vi "Read.vi"(8 "error in (no error)":errorcluster, 9 "Timeout":u32, 10 "Last message":refnum<class "BaseMessage.lvclass">, 11 "StringReader in":refnum<class "StringReader.lvclass">) -> (0 "error out":errorcluster, 1 "isAck?":bool, 2 "Responses":T1[](array[typedef]), 3 "StringReader out":refnum<class "StringReader.lvclass">)   [LabVIEW 2013, in "StringReader.lvclass"]
doc: "Read a message from the remote destination"
uses:
  StringReader.lvclass
  Message/BaseMessage/BaseMessage.lvclass
  response.ctl
  driver_status.ctl
  <vilib>/Utility/error.llb/whitespace.ctl
  StringReader.lvclass/StringReader.ctl
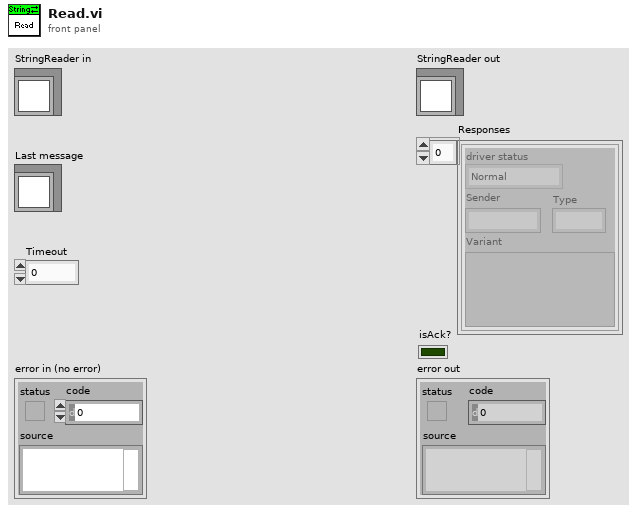
[diagram p1: front panel]
types:
  T1 = typedef "response.ctl" = cluster{"driver status":T2, "Sender":string, "Type":i32, "Variant":variant}
  T2 = typedef "driver_status.ctl" = enum16{"Normal", "Startup", "Connection lost", "Reconnected", "Timeout", "Idle", "Busy"}
  T3 = typedef "whitespace.ctl" = u16
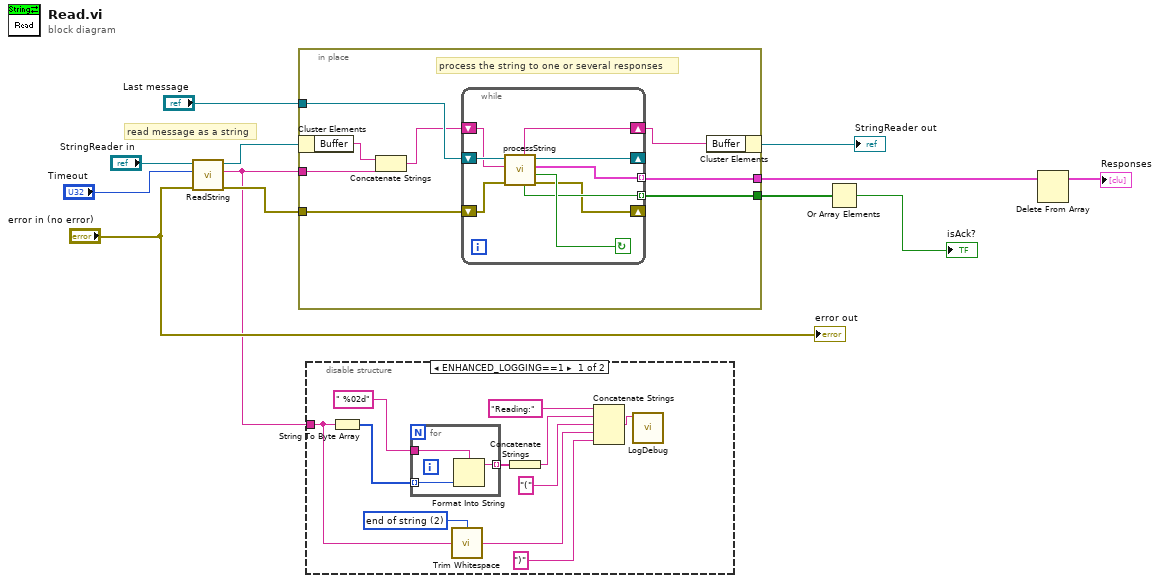
[diagram p0: block diagram]
diagram:
  # "read message as a string"
  n1 = call-dynamic "ReadString.vi"("error in (no error)"="error in (no error)", "Timeout"="Timeout", "StringReader in"="StringReader in") -> ("error out"=w7:errorcluster, "String"=w1:string, "StringReader out"=w6:refnum<class "StringReader.lvclass">)  [unwired: 6 in]
  n2 = in-place "In Place Element Structure" {
    in-place-border: "Last message" -> [w20]
    in-place-border: [w19] -> w4
    in-place-border: [w18] -> w9
    in-place-border: w7 -> [w17]
    in-place-border: w1 -> [w16]
    # "process the string to one or several responses"
    n3 = in-place-cluster #1(w6) -> ("Buffer"=w14:string)
    n4 = Concatenate Strings(w14, w16) -> (w15:string)
    n5 = while {
      shift-right: [w27] -> _
      shift-left: w20 -> [w29]
      tunnel: [w26] -> w19 mode=indexing
      tunnel: [w25] -> w18 mode=indexing
      shift-right: [w23] -> _
      shift-left: w17 -> [w24]
      shift-right: [w21] -> w13
      shift-left: w15 -> [w22]
      stop <- w28 continue-if-true
      n6 = call-dynamic "processString.vi"("error in (no error)"=w24, "Message in"=w22, "Sent message in"=w29) -> ("error out"=w23:errorcluster, "found?"=w28:bool, "response"=w26:T1, "Sent message out"=w27:refnum<class "BaseMessage.lvclass">, "isAck?"=w25:bool, "Remaining buffer"=w21:string)  [unwired: 3 in]
    }
    n7 = in-place-cluster #1("Buffer"=w13) -> (→"StringReader out":refnum<class "StringReader.lvclass">)
  }
  n8 = disable-structure shown="ENHANCED_LOGGING==1" {
    disable-tunnel: w1 -> [w33 _]
    frame condition #0 (active) {
      w30 = T3 2 items=["both", "start of string", "end of string"] ("location (both)")
      n9 = String To Byte Array(string=w33) -> (unsigned byte array=w38:u8[])
      n10 = for {
        tunnel: w38 -> [w43] mode=indexing
        tunnel: [w42] -> w37 mode=indexing
        tunnel: " %02d" ("format string") -> [w41]
        n11 = Format Into String(format string=w41, w43) -> (resulting string=w42:string)  [unwired: 2 in, 1 out]
      }
      n12 = call <vilib>:"Trim Whitespace.vi"("string"=w33, "location (both)"=w30) -> ("trimmed string"=w31:string)
      n13 = Concatenate Strings(w37) -> (w36:string)
      n14 = Concatenate Strings("Reading:" ("string"), w36, "(" ("string"), w31, ")" ("string")) -> (w39:string)
      n15 = call "LogDebug.vi"("Message"=w39) -> ()  [unwired: 7 in, 1 out]
    }
    frame condition #1 {
    }
  }
  n16 = Or Array Elements(Boolean array=w9) -> (logical OR=→"isAck?":bool)
  n17 = Delete From Array(array=w4) -> (array with subset deleted=→"Responses":T1[])  [unwired: 2 in, 1 out]
  "error out" <- "error in (no error)"
